vi "LINC Telemetry Global.vi"(0 "item names in":string[](array[string]), 1 "mode":T3, 2 "target name":string, 5 "item formats in":T2[](array[typedef]), 7 "data in":string, 11 "error in (no error)":errorcluster, 12 "packet name":string, 13 "packet description":string) -> (4 "values out":string[](array[string]), 6 "item formats out":T2[](array[typedef]), 8 "data out":string, 10 "sim ops":T1[](array[typedef])=[{"byte"=0, "mask"=16}, {"byte"=16, "mask"=4}, {"byte"=20, "mask"=12}] {"mask" format="%02x"}, 15 "error out":errorcluster)   [LabVIEW 2018, in "STEPkgDriver_LINC.lvlib"]
uses:
  STEPkgDriver_LINC.lvlib
  LINC Format Prototype.ctl
  LINC Global Prototype.ctl
  LINC Global Mode.ctl
  LINC Sim Ops.ctl
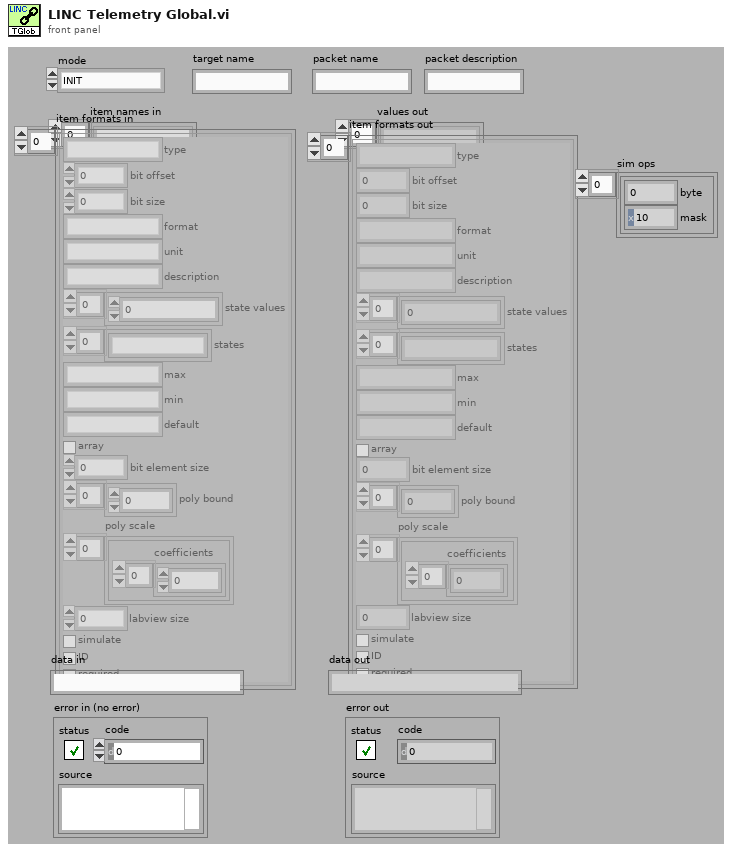
[diagram p1: front panel]
types:
  T1 = typedef "STEPkgDriver_LINC.lvlib/LINC Sim Ops.ctl" = cluster{"byte":i32, "mask":u8}
  T2 = typedef "STEPkgDriver_LINC.lvlib/LINC Format Prototype.ctl" = cluster{"type":string, "bit offset":i32, "bit size":i32, "format":string, "unit":string, "description":string, "state values":i64[], "states":string[], "max":string, "min":string, "default":string, "array":bool, "bit element size":i32, "poly bound":dbl[], "poly scale":cluster{"coefficients":dbl[]}[], "labview size":i32, "simulate":bool, "ID":bool, "required":bool}
  T3 = typedef "STEPkgDriver_LINC.lvlib/LINC Global Mode.ctl" = enum16{"INIT", "CLEAR", "ADD_PKT_HDR", "ADD_PKT", "GET_PKT_NAMES", "GET_PKT_DESC", "GET_PKT_HDR", "GET_PKT", "SET_PKT", "SET_DATA", "SIM_EN", "SIM_DS"}
  T4 = typedef "STEPkgDriver_LINC.lvlib/LINC Global Prototype.ctl" = cluster{"packet names":string[], "packet descriptions":string[], "packet hazardous":bool[], "item names":cluster{"names":string[]}[], "item formats":cluster{"formats":T2[], "sim ops":T1[]}[]}
  T5 = cluster{"item names in":string[], "item formats in":T2[]}
  T6 = cluster{"item formats in":T2[], "sim ops":T1[]}[]
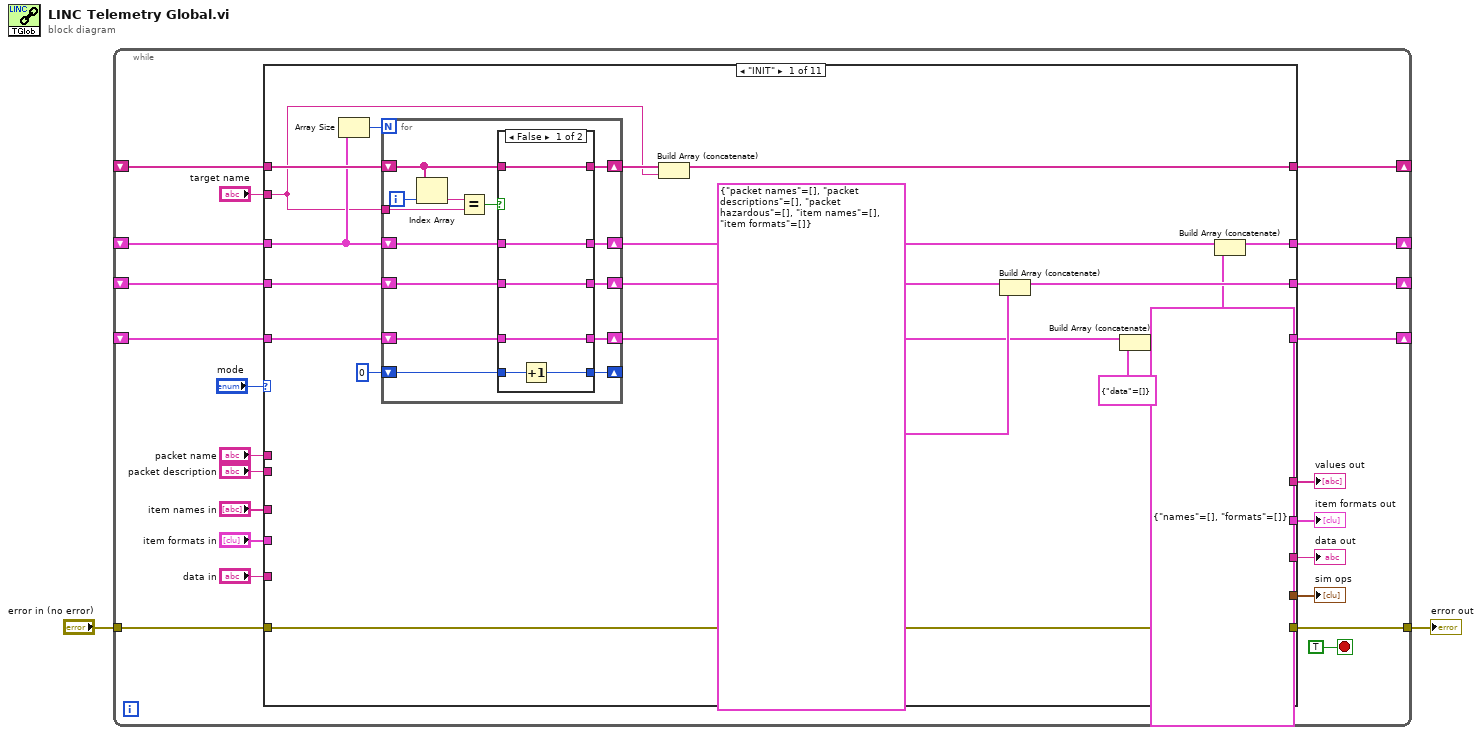
[diagram p0: block diagram]
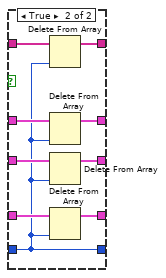
[diagram p2: hidden frame]
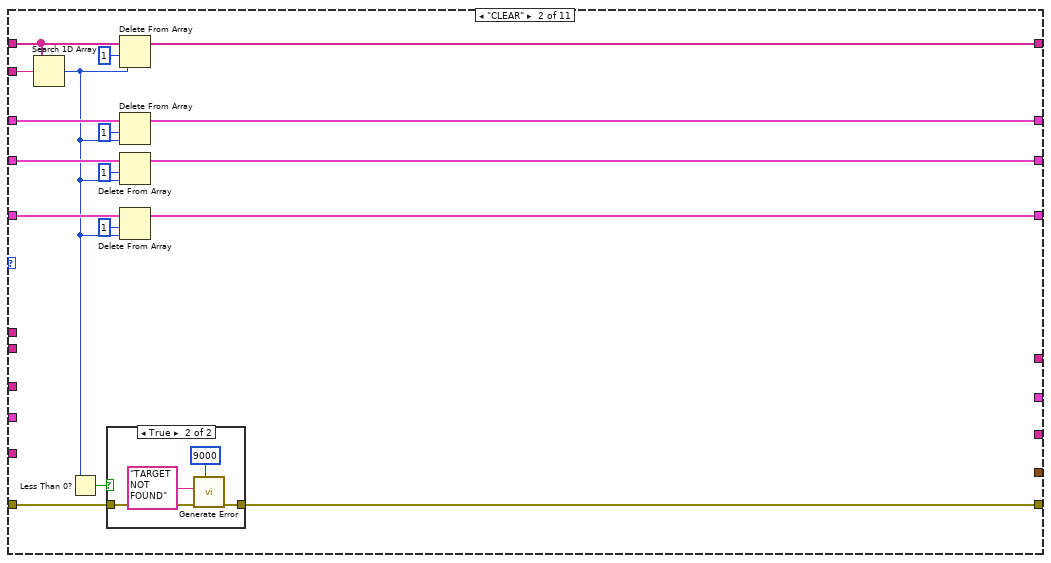
[diagram p3: hidden frame]
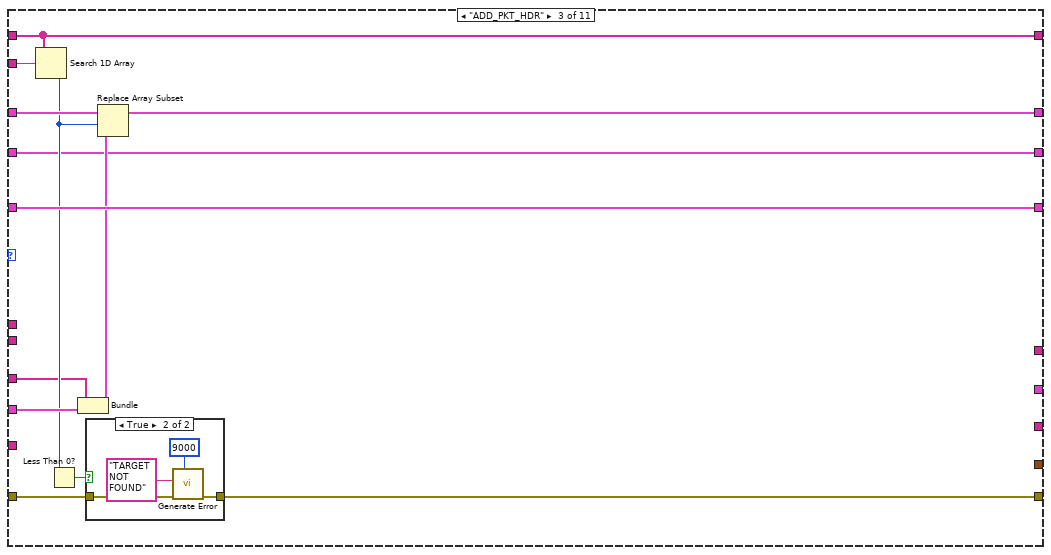
[diagram p5: hidden frame]
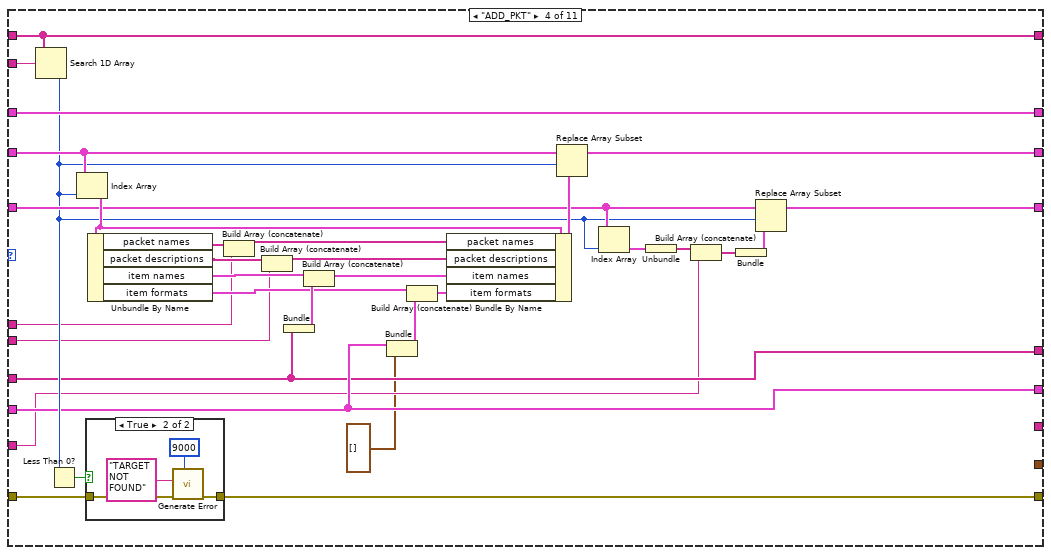
[diagram p7: hidden frame]
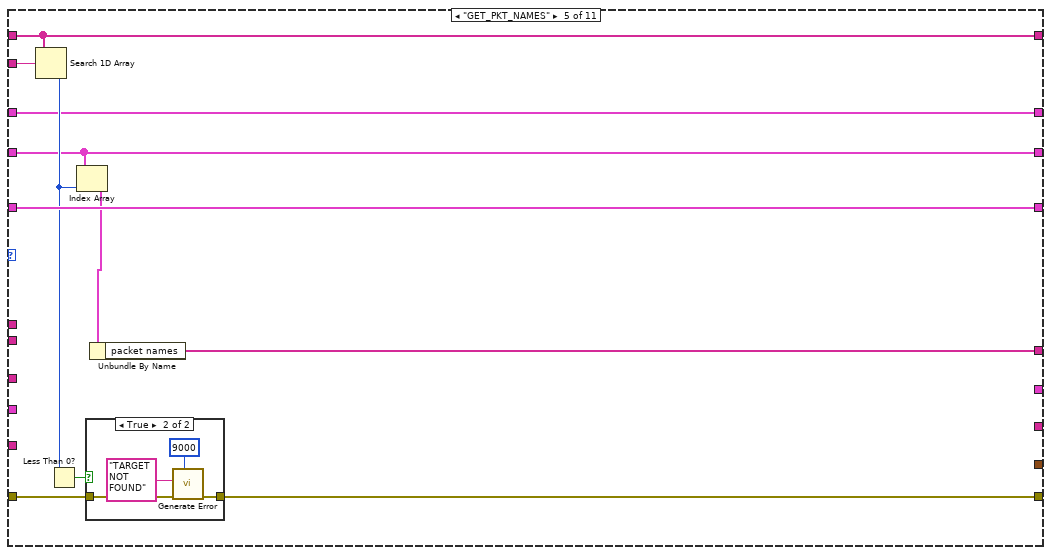
[diagram p9: hidden frame]
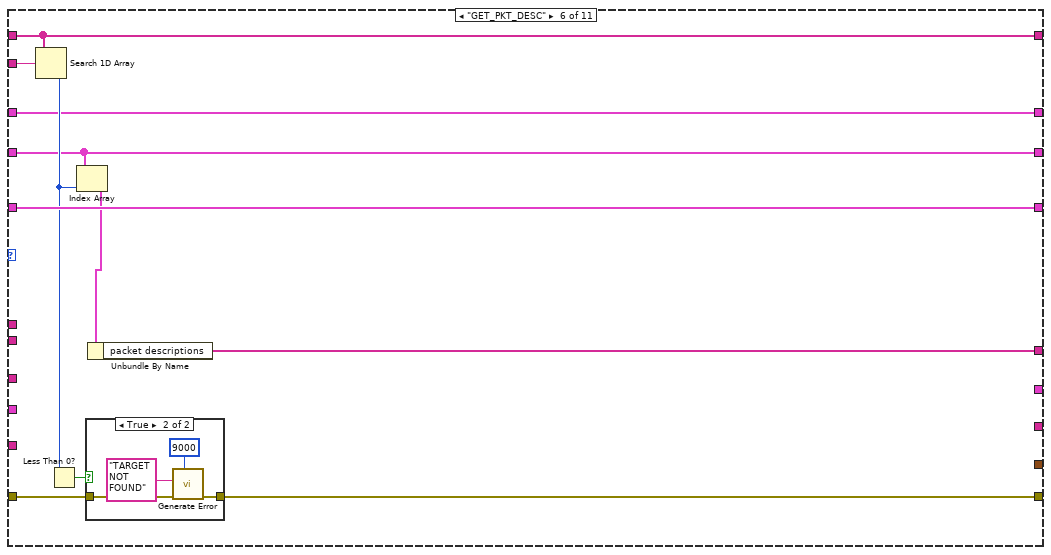
[diagram p11: hidden frame]
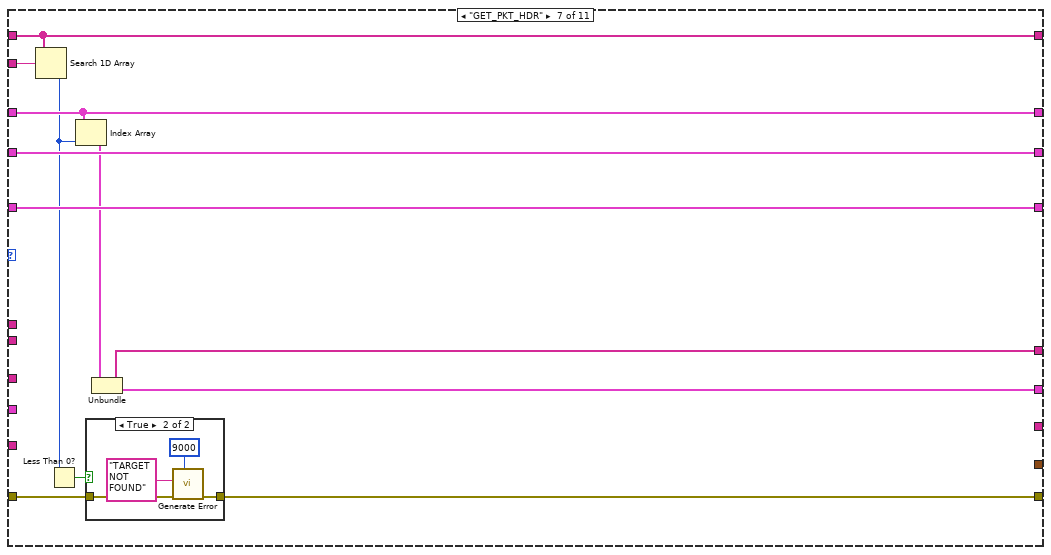
[diagram p13: hidden frame]
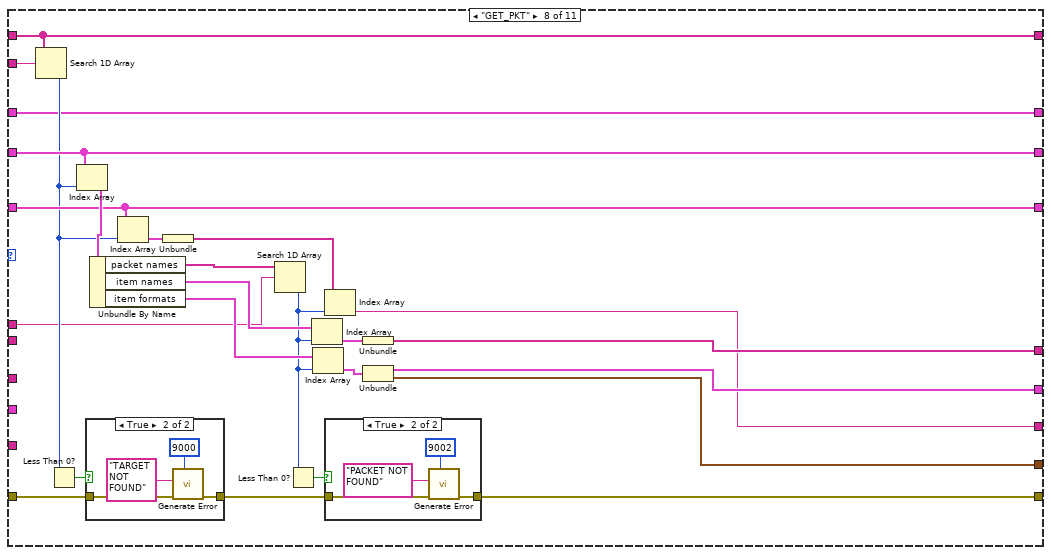
[diagram p15: hidden frame]
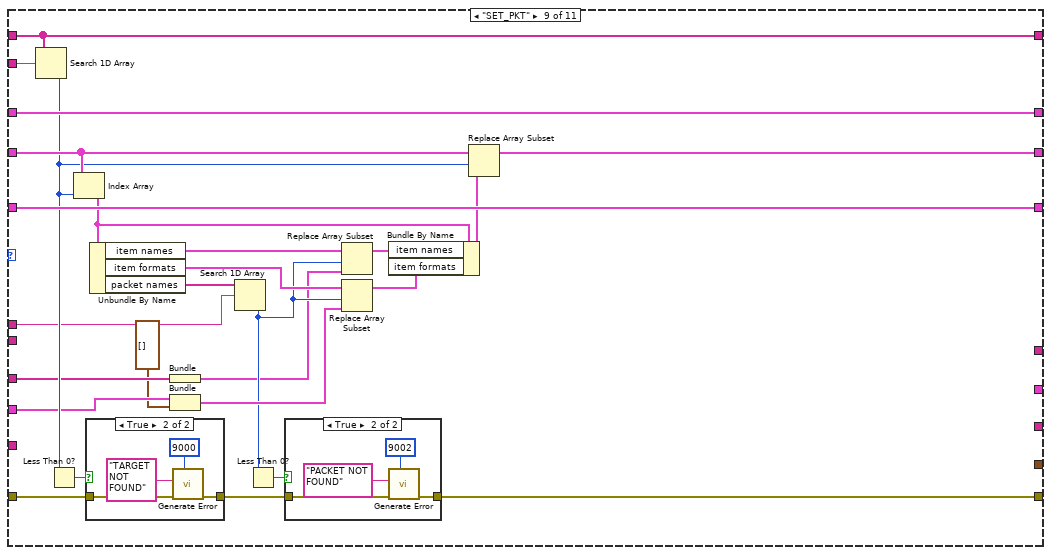
[diagram p18: hidden frame]
diagram:
  n1 = while {
    shift-right: [w22] -> _
    shift-left: _ -> [w23]
    shift-right: [w18] -> _
    shift-left: _ -> [w19]
    shift-right: [w16] -> _
    shift-left: _ -> [w17]
    tunnel: "error in (no error)" -> [w9]
    tunnel: [w8] -> w1
    shift-right: [w7] -> _
    shift-left: _ -> [w6]
    stop <- TRUE stop-if-true
    n2 = case shown="\"INIT\"" "mode" {
      selector: "mode" -> [_ _ _ _ _ _ _ _ _ _ w309]
      tunnel: w23 -> [w33 w88 w107 w145 w161 w177 w194 w224 w260 w287 w336]
      tunnel: [w43 w87 w107 w145 w161 w177 w194 w224 w260 w287 w336] -> w22
      tunnel: "target name" -> [w29 w89 w106 w144 w160 w176 w193 w223 w259 w288 w335]
      tunnel: w19 -> [w31 w84 w96 w130 w152 w168 w192 w214 w250 w286 w322]
      tunnel: [w42 w83 w96 w131 w152 w168 w192 w214 w249 w286 w321] -> w18
      tunnel: w17 -> [w28 w81 w101 w125 w159 w175 w189 w208 w252 w284 w313]
      tunnel: [w41 w80 w101 w126 w159 w175 w189 w208 w252 w285 w313] -> w16
      tunnel: "item names in" -> [_ _ w95 w117 _ _ _ _ w241 _ w326]
      tunnel: "item formats in" -> [_ _ w102 w118 _ _ _ _ w243 _ _]
      tunnel: [_ _ _ w117 w153 w169 w183 w216 _ _ w315] -> w13
      tunnel: [_ _ _ w118 _ _ w184 w215 _ _ w303] -> w12
      tunnel: [_ _ _ _ _ _ _ w204 _ _ w310] -> w11
      tunnel: "data in" -> [_ _ _ w116 _ _ _ _ _ w280 _]
      tunnel: w9 -> [w38 w78 w104 w128 w156 w172 w190 w212 w256 w276 w329]
      tunnel: [w38 w77 w103 w121 w154 w170 w185 w209 w253 w275 w317] -> w8
      tunnel: w6 -> [w30 w75 w100 w120 w151 w167 w188 w203 w251 w272 w306]
      tunnel: [w37 w73 w99 w120 w151 w167 w188 w203 w251 w272 w306] -> w7
      tunnel: "packet name" -> [_ _ _ w115 _ _ _ w202 w236 w271 w304]
      tunnel: "packet description" -> [_ _ _ w114 _ _ _ _ _ _ _]
      tunnel: [_ _ _ _ _ _ _ w200 _ _ _] -> w3
      frame "INIT" {
        n3 = Array Size(array=w30) -> (size(s)=w35:i32)
        n4 = for {
          N: w35 -> [_]
          shift-right: [w50] -> w32
          shift-left: w33 -> [w56]
          shift-right: [w49] -> w27
          shift-left: w30 -> [w55]
          shift-right: [w48] -> w26
          shift-left: w31 -> [w54]
          tunnel: w29 -> [w52]
          shift-right: [w46] -> _
          shift-left: 0 -> [w47]
          shift-right: [w44] -> w25
          shift-left: w28 -> [w45]
          i -> [w57]
          n5 = Index Array(array=w56, index=w57) -> (element=w53:string)
          n6 = Equal?(x=w53, y=w52) -> (x = y?=w51:bool)
          n7 = case shown="False" w51 {
            tunnel: w56 -> [w63 w72]
            tunnel: w55 -> [w62 w70]
            tunnel: w54 -> [w61 w69]
            tunnel: [w63 w71] -> w50
            tunnel: [w62 w68] -> w49
            tunnel: [w61 w67] -> w48
            tunnel: w47 -> [w60 w65]
            tunnel: [w59 w65] -> w46
            tunnel: w45 -> [w58 w66]
            tunnel: [w58 w64] -> w44
            frame False {
              n8 = Increment(x=w60) -> (x+1=w59:i32)
            }
            frame True {
              n9 = Delete From Array(array=w72, index=w65) -> (array with subset deleted=w71:string[])  [unwired: 1 in, 1 out]
              n10 = Delete From Array(array=w70, index=w65) -> (array with subset deleted=w68:cluster{"names":string[], "formats":T2[]}[])  [unwired: 1 in, 1 out]
              n11 = Delete From Array(array=w69, index=w65) -> (array with subset deleted=w67:T4[])  [unwired: 1 in, 1 out]
              n12 = Delete From Array(array=w66, index=w65) -> (array with subset deleted=w64:cluster{"data":string[]}[])  [unwired: 1 in, 1 out]
            }
          }
        }
        n13 = Build Array (concatenate)(w32, w29) -> (w43:string[])
        n14 = Build Array (concatenate)(w26, T4 {"packet names"=[], "packet descriptions"=[], "packet hazardous"=[], "item names"=[], "item formats"=[]} ("housekeeping")) -> (w42:T4[])
        n15 = Build Array (concatenate)(w25, cluster{"data":string[]} {"data"=[]} ("data")) -> (w41:cluster{"data":string[]}[])
        n16 = Build Array (concatenate)(w27, cluster{"names":string[], "formats":T2[]} {"names"=[], "formats"=[]}) -> (w37:cluster{"names":string[], "formats":T2[]}[])
      }
      frame "CLEAR" {
        n17 = Search 1D Array(1D array=w88, element=w89) -> (index of element=w74:i32)  [unwired: 1 in]
        n18 = Less Than 0?(x=w74) -> (x < 0?=w79:bool)
        n19 = case shown="True" w79 {
          tunnel: w78 -> [w90 w94]
          tunnel: [w90 w93] -> w77
          frame False {
          }
          frame True {
            n20 = call "Generate Error.vi"("error code (-1301)"=9000, "error in"=w94, "description"="TARGET NOT FOUND") -> ("error out"=w93:errorcluster)  [unwired: 8 in]
          }
        }
        n21 = Delete From Array(array=w88, length=1, index=w74) -> (array with subset deleted=w87:string[])  [unwired: 1 out]
        n22 = Delete From Array(array=w75, length=1, index=w74) -> (array with subset deleted=w73:cluster{"names":string[], "formats":T2[]}[])  [unwired: 1 out]
        n23 = Delete From Array(array=w84, length=1, index=w74) -> (array with subset deleted=w83:T4[])  [unwired: 1 out]
        n24 = Delete From Array(array=w81, length=1, index=w74) -> (array with subset deleted=w80:cluster{"data":string[]}[])  [unwired: 1 out]
      }
      frame "ADD_PKT_HDR" {
        n25 = Search 1D Array(1D array=w107, element=w106) -> (index of element=w98:i32)  [unwired: 1 in]
        n26 = Less Than 0?(x=w98) -> (x < 0?=w105:bool)
        n27 = Bundle("item names in"=w95, "item formats in"=w102) -> (w97:T5)  [unwired: 1 in]
        n28 = case shown="True" w105 {
          tunnel: w104 -> [w108 w112]
          tunnel: [w108 w111] -> w103
          frame False {
          }
          frame True {
            n29 = call "Generate Error.vi"("error code (-1301)"=9000, "error in"=w112, "description"="TARGET NOT FOUND") -> ("error out"=w111:errorcluster)  [unwired: 8 in]
          }
        }
        n30 = Replace Array Subset(array=w100, new element=w97, index=w98) -> (w99:cluster{"names":string[], "formats":T2[]}[])
      }
      frame "ADD_PKT" {
        n31 = Search 1D Array(1D array=w145, element=w144) -> (index of element=w119:i32)  [unwired: 1 in]
        n32 = Less Than 0?(x=w119) -> (x < 0?=w129:bool)
        n33 = Index Array(array=w130, index=w119) -> (element=w137:T4)
        n34 = case shown="True" w129 {
          tunnel: w128 -> [w146 w150]
          tunnel: [w146 w149] -> w121
          frame False {
          }
          frame True {
            n35 = call "Generate Error.vi"("error code (-1301)"=9000, "error in"=w150, "description"="TARGET NOT FOUND") -> ("error out"=w149:errorcluster)  [unwired: 8 in]
          }
        }
        n36 = Unbundle By Name(w137) -> ("packet names"=w143:string[], "packet descriptions"=w142:string[], "item names"=w141:cluster{"names":string[]}[], "item formats"=w139:cluster{"formats":T2[], "sim ops":T1[]}[])
        n37 = Build Array (concatenate)(w143, w115) -> (w136:string[])
        n38 = Build Array (concatenate)(w142, w114) -> (w135:string[])
        n39 = Bundle("item names in"=w117) -> (w140:cluster{"item names in":string[]})  [unwired: 1 in]
        n40 = Build Array (concatenate)(w141, w140) -> (w134:cluster{"item names in":string[]}[])
        n41 = Bundle("item formats in"=w118, "sim ops"=T1[] []) -> (w138:cluster{"item formats in":T2[], "sim ops":T1[]})  [unwired: 1 in]
        n42 = Build Array (concatenate)(w139, w138) -> (w133:T6)
        n43 = Bundle By Name(cluster=w137, "packet names"=w136, "packet descriptions"=w135, "item names"=w134, "item formats"=w133) -> (w132:T4)
        n44 = Replace Array Subset(array=w130, new element=w132, index=w119) -> (w131:T4[])
        n45 = Index Array(array=w125, index=w119) -> (element=w124:cluster{"data":string[]})
        n46 = Unbundle(w124) -> ("data"=w123:string[])
        n47 = Build Array (concatenate)(w123, w116) -> (w122:string[])
        n48 = Bundle(w122) -> (w127:cluster{string[]})  [unwired: 1 in]
        n49 = Replace Array Subset(array=w125, new element=w127, index=w119) -> (w126:cluster{"data":string[]}[])
      }
      frame "GET_PKT_NAMES" {
        n50 = Search 1D Array(1D array=w161, element=w160) -> (index of element=w155:i32)  [unwired: 1 in]
        n51 = Less Than 0?(x=w155) -> (x < 0?=w157:bool)
        n52 = Index Array(array=w152, index=w155) -> (element=w158:T4)
        n53 = case shown="True" w157 {
          tunnel: w156 -> [w162 w166]
          tunnel: [w162 w165] -> w154
          frame False {
          }
          frame True {
            n54 = call "Generate Error.vi"("error code (-1301)"=9000, "error in"=w166, "description"="TARGET NOT FOUND") -> ("error out"=w165:errorcluster)  [unwired: 8 in]
          }
        }
        n55 = Unbundle By Name(w158) -> ("packet names"=w153:string[])
      }
      frame "GET_PKT_DESC" {
        n56 = Search 1D Array(1D array=w177, element=w176) -> (index of element=w171:i32)  [unwired: 1 in]
        n57 = Less Than 0?(x=w171) -> (x < 0?=w173:bool)
        n58 = Index Array(array=w168, index=w171) -> (element=w174:T4)
        n59 = case shown="True" w173 {
          tunnel: w172 -> [w178 w182]
          tunnel: [w178 w181] -> w170
          frame False {
          }
          frame True {
            n60 = call "Generate Error.vi"("error code (-1301)"=9000, "error in"=w182, "description"="TARGET NOT FOUND") -> ("error out"=w181:errorcluster)  [unwired: 8 in]
          }
        }
        n61 = Unbundle By Name(w174) -> ("packet descriptions"=w169:string[])
      }
      frame "GET_PKT_HDR" {
        n62 = Search 1D Array(1D array=w194, element=w193) -> (index of element=w187:i32)  [unwired: 1 in]
        n63 = Less Than 0?(x=w187) -> (x < 0?=w191:bool)
        n64 = Index Array(array=w188, index=w187) -> (element=w186:cluster{"names":string[], "formats":T2[]})
        n65 = case shown="True" w191 {
          tunnel: w190 -> [w195 w199]
          tunnel: [w195 w198] -> w185
          frame False {
          }
          frame True {
            n66 = call "Generate Error.vi"("error code (-1301)"=9000, "error in"=w199, "description"="TARGET NOT FOUND") -> ("error out"=w198:errorcluster)  [unwired: 8 in]
          }
        }
        n67 = Unbundle(w186) -> ("names"=w183:string[], "formats"=w184:T2[])
      }
      frame "GET_PKT" {
        n68 = Search 1D Array(1D array=w224, element=w223) -> (index of element=w207:i32)  [unwired: 1 in]
        n69 = Less Than 0?(x=w207) -> (x < 0?=w213:bool)
        n70 = Index Array(array=w214, index=w207) -> (element=w222:T4)
        n71 = case shown="True" w213 {
          tunnel: w212 -> [w230 w234]
          tunnel: [w230 w233] -> w210
          frame False {
          }
          frame True {
            n72 = call "Generate Error.vi"("error code (-1301)"=9000, "error in"=w234, "description"="TARGET NOT FOUND") -> ("error out"=w233:errorcluster)  [unwired: 8 in]
          }
        }
        n73 = Unbundle By Name(w222) -> ("packet names"=w221:string[], "item names"=w220:cluster{"names":string[]}[], "item formats"=w219:cluster{"formats":T2[], "sim ops":T1[]}[])
        n74 = Index Array(array=w208, index=w207) -> (element=w206:cluster{"data":string[]})
        n75 = Unbundle(w206) -> ("data"=w205:string[])
        n76 = Search 1D Array(1D array=w221, element=w202) -> (index of element=w201:i32)  [unwired: 1 in]
        n77 = Less Than 0?(x=w201) -> (x < 0?=w211:bool)
        n78 = Index Array(array=w220, index=w201) -> (element=w218:cluster{"names":string[]})
        n79 = Index Array(array=w219, index=w201) -> (element=w217:cluster{"formats":T2[], "sim ops":T1[]})
        n80 = Index Array(array=w205, index=w201) -> (element=w204:string)
        n81 = case shown="True" w211 {
          tunnel: w210 -> [w225 w229]
          tunnel: [w225 w228] -> w209
          frame False {
          }
          frame True {
            n82 = call "Generate Error.vi"("error code (-1301)"=9002, "error in"=w229, "description"="PACKET NOT FOUND") -> ("error out"=w228:errorcluster)  [unwired: 8 in]
          }
        }
        n83 = Unbundle(w218) -> ("names"=w216:string[])
        n84 = Unbundle(w217) -> ("formats"=w215:T2[], "sim ops"=w200:T1[])
      }
      frame "SET_PKT" {
        n85 = Search 1D Array(1D array=w260, element=w259) -> (index of element=w248:i32)  [unwired: 1 in]
        n86 = Less Than 0?(x=w248) -> (x < 0?=w257:bool)
        n87 = Index Array(array=w250, index=w248) -> (element=w246:T4)
        n88 = case shown="True" w257 {
          tunnel: w256 -> [w266 w270]
          tunnel: [w266 w269] -> w254
          frame False {
          }
          frame True {
            n89 = call "Generate Error.vi"("error code (-1301)"=9000, "error in"=w270, "description"="TARGET NOT FOUND") -> ("error out"=w269:errorcluster)  [unwired: 8 in]
          }
        }
        n90 = Unbundle By Name(w246) -> ("item names"=w240:cluster{"names":string[]}[], "item formats"=w247:cluster{"formats":T2[], "sim ops":T1[]}[], "packet names"=w258:string[])
        n91 = Bundle("item names in"=w241) -> (w237:cluster{"item names in":string[]})  [unwired: 1 in]
        n92 = Bundle("item formats in"=w243, "sim ops"=T1[] []) -> (w242:cluster{"item formats in":T2[], "sim ops":T1[]})  [unwired: 1 in]
        n93 = Search 1D Array(1D array=w258, element=w236) -> (index of element=w238:i32)  [unwired: 1 in]
        n94 = Less Than 0?(x=w238) -> (x < 0?=w255:bool)
        n95 = case shown="True" w255 {
          tunnel: w254 -> [w261 w265]
          tunnel: [w261 w264] -> w253
          frame False {
          }
          frame True {
            n96 = call "Generate Error.vi"("error code (-1301)"=9002, "error in"=w265, "description"="PACKET NOT FOUND") -> ("error out"=w264:errorcluster)  [unwired: 8 in]
          }
        }
        n97 = Replace Array Subset(array=w240, new element=w237, index=w238) -> (w239:cluster{"names":string[]}[])
        n98 = Replace Array Subset(array=w247, new element=w242, index=w238) -> (w245:cluster{"formats":T2[], "sim ops":T1[]}[])
        n99 = Bundle By Name(cluster=w246, "item names"=w239, "item formats"=w245) -> (w244:T4)
        n100 = Replace Array Subset(array=w250, new element=w244, index=w248) -> (w249:T4[])
      }
      frame "SET_DATA" {
        n101 = Search 1D Array(1D array=w287, element=w288) -> (index of element=w274:i32)  [unwired: 1 in]
        n102 = Less Than 0?(x=w274) -> (x < 0?=w279:bool)
        n103 = Index Array(array=w286, index=w274) -> (element=w291:T4)
        n104 = case shown="True" w279 {
          tunnel: w276 -> [w297 w301]
          tunnel: [w297 w300] -> w277
          frame False {
          }
          frame True {
            n105 = call "Generate Error.vi"("error code (-1301)"=9000, "error in"=w301, "description"="TARGET NOT FOUND") -> ("error out"=w300:errorcluster)  [unwired: 8 in]
          }
        }
        n106 = Unbundle By Name(w291) -> ("packet names"=w290:string[])
        n107 = Index Array(array=w284, index=w274) -> (element=w289:cluster{"data":string[]})
        n108 = Unbundle(w289) -> ("data"=w283:string[])
        n109 = Search 1D Array(1D array=w290, element=w271) -> (index of element=w273:i32)  [unwired: 1 in]
        n110 = Less Than 0?(x=w273) -> (x < 0?=w278:bool)
        n111 = Replace Array Subset(array=w283, new element=w280, index=w273) -> (w282:string[])
        n112 = case shown="True" w278 {
          tunnel: w277 -> [w292 w296]
          tunnel: [w292 w295] -> w275
          frame False {
          }
          frame True {
            n113 = call "Generate Error.vi"("error code (-1301)"=9002, "error in"=w296, "description"="PACKET NOT FOUND") -> ("error out"=w295:errorcluster)  [unwired: 8 in]
          }
        }
        n114 = Bundle("data"=w282) -> (w281:cluster{"data":string[]})  [unwired: 1 in]
        n115 = Replace Array Subset(array=w284, new element=w281, index=w274) -> (w285:cluster{"data":string[]}[])
      }
      frame "SIM_EN", "SIM_DS" {
        n116 = Equal?(x=w309, y=LINC_Global_Mode."SIM_EN" ("mode")) -> (x = y?=w308:bool)
        n117 = Search 1D Array(1D array=w336, element=w335) -> (index of element=w312:i32)  [unwired: 1 in]
        n118 = Less Than 0?(x=w312) -> (x < 0?=w330:bool)
        n119 = Index Array(array=w322, index=w312) -> (element=w320:T4)
        n120 = case shown="True" w330 {
          tunnel: w329 -> [w358 w362]
          tunnel: [w358 w361] -> w327
          frame False {
          }
          frame True {
            n121 = call "Generate Error.vi"("error code (-1301)"=9000, "error in"=w362, "description"="TARGET NOT FOUND") -> ("error out"=w361:errorcluster)  [unwired: 8 in]
          }
        }
        n122 = Unbundle By Name(w320) -> ("packet names"=w334:string[], "item names"=w333:cluster{"names":string[]}[], "item formats"=w323:cluster{"formats":T2[], "sim ops":T1[]}[])
        n123 = Index Array(array=w313, index=w312) -> (element=w314:cluster{"data":string[]})
        n124 = Unbundle(w314) -> ("data"=w311:string[])
        n125 = Search 1D Array(1D array=w334, element=w304) -> (index of element=w307:i32)  [unwired: 1 in]
        n126 = Less Than 0?(x=w307) -> (x < 0?=w328:bool)
        n127 = Index Array(array=w311, index=w307) -> (element=w310:string)
        n128 = Index Array(array=w333, index=w307) -> (element=w332:cluster{"names":string[]})
        n129 = Index Array(array=w323, index=w307) -> (element=w331:cluster{"formats":T2[], "sim ops":T1[]})
        n130 = case shown="True" w328 {
          tunnel: w327 -> [w353 w357]
          tunnel: [w353 w356] -> w318
          frame False {
          }
          frame True {
            n131 = call "Generate Error.vi"("error code (-1301)"=9002, "error in"=w357, "description"="PACKET NOT FOUND") -> ("error out"=w356:errorcluster)  [unwired: 8 in]
          }
        }
        n132 = Unbundle(w332) -> ("names"=w315:string[])
        n133 = Unbundle(w331) -> ("formats"=w325:T2[])  [unwired: 1 out]
        n134 = for {
          tunnel: w315 -> [w347]
          tunnel: w326 -> [w346] mode=indexing
          shift-right: [w343] -> w303
          shift-left: w325 -> [w344]
          shift-right: [w341] -> w317
          shift-left: w318 -> [w340]
          tunnel: w308 -> [w337]
          n135 = Search 1D Array(1D array=w347, element=w346) -> (index of element=w339:i32)  [unwired: 1 in]
          n136 = Less Than 0?(x=w339) -> (x < 0?=w338:bool)
          n137 = Index Array(array=w344, index=w339) -> (element=w345:T2)
          n138 = Bundle By Name(cluster=w345, "simulate"=w337) -> (w342:T2)
          n139 = Replace Array Subset(array=w344, new element=w342, index=w339) -> (w343:T2[])
          n140 = case shown="True" w338 {
            tunnel: w340 -> [w348 w352]
            tunnel: [w348 w351] -> w341
            frame False {
            }
            frame True {
              n141 = call "Generate Error.vi"("error code (-1301)"=9003, "error in"=w352, "description"="ITEM NOT FOUND") -> ("error out"=w351:errorcluster)  [unwired: 8 in]
            }
          }
        }
        n142 = call "LINC Compile Sim Ops.vi"("item formats"=w303) -> ("sim ops"=w302:T1[])
        n143 = Bundle("formats"=w303, "sim ops"=w302) -> (w324:cluster{"formats":T2[], "sim ops":T1[]})  [unwired: 1 in]
        n144 = Replace Array Subset(array=w323, new element=w324, index=w307) -> (w316:cluster{"formats":T2[], "sim ops":T1[]}[])
        n145 = Bundle By Name(cluster=w320, "item formats"=w316) -> (w319:T4)
        n146 = Replace Array Subset(array=w322, new element=w319, index=w312) -> (w321:T4[])
      }
    }
    "values out" <- w13
    "item formats out" <- w12
    "data out" <- w11
    "sim ops" <- w3
  }
  "error out" <- w1
